vi "UDP-Client.vi"() -> ()   [LabVIEW 2020]
doc: "The UDP protocol differs from TCP in that there is no error-checking with the packets of information that are sent, and thus no guarantee whatsoever that an intended recipient will actually receive a given piece of data.\n\nUDP does offer the ability to \"broadcast\" data across a network--simply specify an IP Address of all ones (255.255.255.255) to attempt to broadcast information network-wide. Keep in mind that routers and other network hardware will generally refuse to forward the broadcast beyond certain points, so the extent of the broadcast will in practice be limited."
panel:
  out "Received Data":dbl(graph)
  in  "Stop":bool
  # "Overview: Demonstrates the use of the UDP functions to receive data over a UDP connection.\nInstructions:\n1. Ensure Simple UDP - Sender.vi is already running.\n2. Run the VI.\n3. Click Stop to stop the VI."
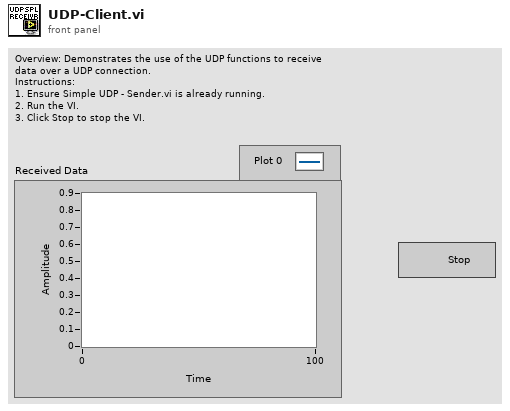
[diagram p1: front panel]
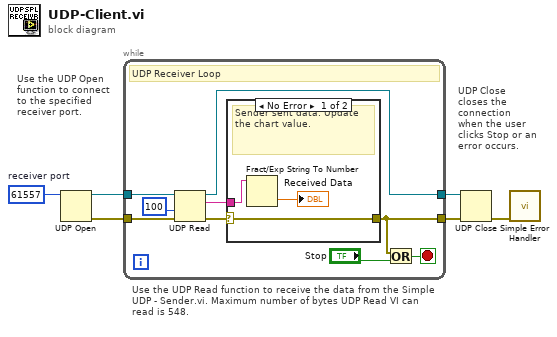
[diagram p0: block diagram]
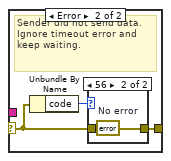
[diagram p2: hidden frame]
diagram:
  w1 = u16 61557  # receiver port
  # "UDP Close closes the connection when the user clicks Stop or an error occurs."
  # "Use the UDP Open function to connect to the specified receiver port."
  # "Use the UDP Read function to receive the data from the Simple UDP - Sender.vi. Maximum number of bytes UDP Read VI can read is 548."
  n1 = UDP Open(11:w1) -> (port=w2:refnum<k16>, 0:w3:errorcluster)  [unwired: 4 in, 1 out]
  n2 = while {
    tunnel: w2 -> [w15]
    tunnel: [w7] -> w6
    tunnel: w3 -> [w12]
    tunnel: [w8] -> w4
    stop <- w13 stop-if-true
    # "UDP Receiver Loop"
    n3 = UDP Read(connection ID=w15, timeout ms (25000)=100, 8:w12) -> (data out=w10:string, error out=w9:errorcluster, 3:w7:refnum<k16>)  [unwired: 3 out]
    n4 = case shown="No Error" w9 {
      selector: w9 -> [w16 w20]
      tunnel: w10 -> [w18 _]
      tunnel: [w16 w19] -> w8
      frame No Error {
        # "Sender sent data. Update the chart value."
        n5 = Fract/Exp String To Number(string=w18) -> (number=→"Received Data":dbl)  [unwired: 3 in, 1 out]
      }
      frame Error {
        # "Sender did not send data. Ignore timeout error and keep waiting."
        n6 = Unbundle By Name(w20) -> ("code"=w21:i32)
        n7 = case shown="56" w21 {
          tunnel: w20 -> [w22 _]
          tunnel: [w22 w23] -> w19
          frame Default {
          }
          frame 56 {
            w23 = errorcluster {"status"=FALSE, "code"=0, "source"=""}  # No error
          }
        }
      }
    }
    n8 = Or(x=w8, y="Stop") -> (x .or. y?=w13:bool)
  }
  n9 = UDP Close(connection ID=w6, 8:w4) -> (error out=w5:errorcluster)  [unwired: 1 out]
  n10 = call <vilib>:"Simple Error Handler.vi"("error in (no error)"=w5) -> ()  [unwired: 1 in, 8 out]
